vi "PH_Timing.PC link BNC Channel Infos.vi"(0 "i ref in":refnum<vi>, 1 "data":i8[](array[numeric]), 2 "Service Name":string="N/A", 3 "typeDescriptor":string="D:N", 4 "no link":bool, 5 "error in":errorcluster) -> (14 "i ref out":refnum<vi>, 19 "error out":errorcluster)   [LabVIEW 2014, in "PH_Timing.lvlib"]
doc: "This VI writes the incoming information to own attributes and sets GUI elements."
uses:
  PH_Timing.lvlib
  PH_Basics/PH_Common/PH_Common.lvlib
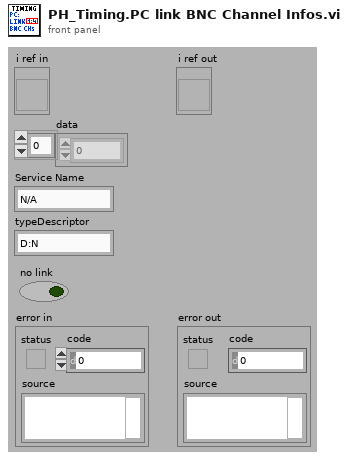
[diagram p1: front panel]
types:
  T1 = typedef "PH_Timing.lvlib/PH_Timing.i attribute.ctl" = cluster{"Sequencer":cluster{"linked?":bool, "Proc State":string, "Ref State":refnum<vi>}, "Gate Generator":cluster{"GD":cluster{"Device Status":T2, "linked?":bool}, "Settings":T3, "GUI Ref":refnum<vi>}, "Interlock Bypass":cluster{"Instancename":string, "Switch linked?":bool, "Device Status":T2, "Ref Status":refnum<vi>}, "Roughtuner":cluster{"Settings":T4, "GUI Ref":refnum<vi>, "GD":cluster{"Device Status":T2, "linked?":bool}}, "0,5Hz Gater":cluster{"Settings":T5, "GUI Ref":refnum<vi>, "GD":cluster{"Device Status":T2, "linked?":bool}}, "Slow Trigger":cluster{"Settings":T6, "GUI Ref":refnum<vi>, "Service ID Delay":i32, "Service ID Ext Trig":i32, "Wanted Settings":T6}, "Timing Mode":cluster{"Mode":T7, "GUI Ref":refnum<vi>, "Service ID T2":i32, "Service ID Mode":i32, "Wanted Mode":T7}, "ns Generator":cluster{"Settings":T8, "ns Generator Settings":refnum<vi>, "GD":cluster{"Device Status":T2, "linked?":bool}}, "Phase FEs":cluster{"Settings":T11, "GUI Ref":refnum<vi>, "Service ID Phase":i32, "Wanted Settings":T11}, "GD GUI Refs":refnum<vi>[], "Heads":T12[], "GUI Ref Delete":refnum<vi>}
  T2 = typedef "PH_StatusHandler.lvlib/PH_StatusHandler.Status.ctl" = i16
  T3 = typedef "PH_Timing.lvlib/PH_Timing.GateGen.ctl" = cluster{"Instance":string, "Channel Gate":i32, "Channel T2":i32, "Width Gate":dbl, "Width T2":dbl, "Delay Gate":dbl, "Delay T2":dbl, "Gate activ":bool, "T2 activ":bool, "System Mode":enum16{"Normal", "Single", "Burst", "Duty Cycle"}}
  T4 = typedef "PH_Timing.lvlib/PH_Timing.Roughtuner.ctl" = cluster{"Instance":string, "Phase PHELIX / UNILAC":cluster{"Channel":u16, "relative to":u16, "Delay [ms]":dbl}, "Pulse Length":cluster{"Channel":u16, "relative to":u16, "Delay [ms]":dbl}, "Trigger":cluster{"externally?":bool, "Rate [Hz]":dbl}}
  T5 = typedef "PH_Timing.lvlib/PH_Timing.0.5HzGater.ctl" = cluster{"Instance":string, "Channel ns FE Delay":i32, "Channel 0.5Hz":i32, "Width ns FE Delay":dbl, "Width 0.5Hz":dbl, "Delay ns FE Delay":dbl, "Delay 0.5Hz":dbl, "ns FE Delay active":bool, "0.5Hz activ":bool, "ns FE Delay inverted":bool, "0.5Hz inverted":bool}
  T6 = typedef "PH_Timing.lvlib/PH_Timing.Slow Trigger Settings.ctl" = cluster{"Delay":dbl, "externally triggered?":bool}
  T7 = typedef "PH_Timing.lvlib/PH_Timing.Timing Mode.ctl" = cluster{"T2":i16, "Modeselector":enum32{"10 Hz", "0.5 Hz", "Shot"}}
  T8 = typedef "PH_Timing.lvlib/PH_Timing.ns Generator.ctl" = cluster{"Instance":string, "Phase fs / ns FE":cluster{"Channel":T9, "Settings":T10}}
  T9 = typedef "Stanford Research DG645 - Driver.lvlib/Channel.ctl" = i32
  T10 = typedef "PH_SRDG645.lvlib/PH_SRDG645.Channel Settings.ctl" = cluster{"Delay [s]":dbl, "relative to":i32}
  T11 = typedef "PH_Timing.lvlib/PH_Timing.Phase FEs.ctl" = cluster{"Phase":dbl}
  T12 = typedef "PH_Timing.lvlib/PH_Timing.PU Data.ctl" = cluster{"linked?":bool, "Data":T13, "GD":cluster{"Device Status":T2, "linked?":bool}, "GUI Ref":refnum<vi>, "PU":T14}
  T13 = typedef "PH_Timing.lvlib/PH_Timing.PU Info.ctl" = cluster{"Act CH?":bool, "GD":string, "CH":i32, "Delay":dbl, "active":bool, "in Use?":bool}
  T14 = typedef "PH_PP_Common.lvlib/PH_PP_Common.PUs.ctl" = enum16{"no Info", "PA-19mm-1", "PA-19mm-2", "PA-45mm-PILC", "PA-45mm-MAIN", "MA-PU-1", "MA-PU-2", "MA-PU-3", "MA-PU-4", "MA-PU-5", "MA-PU-6", "MA-FR", "MA-PILC", "PA-45mm-DP"}
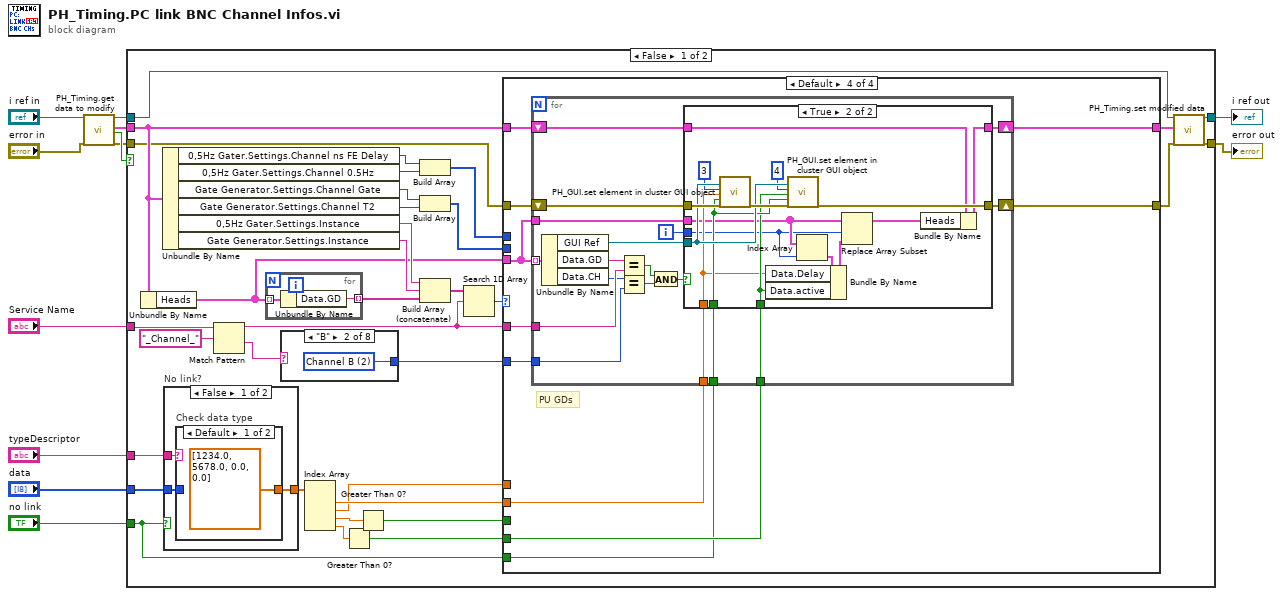
[diagram p0: block diagram]
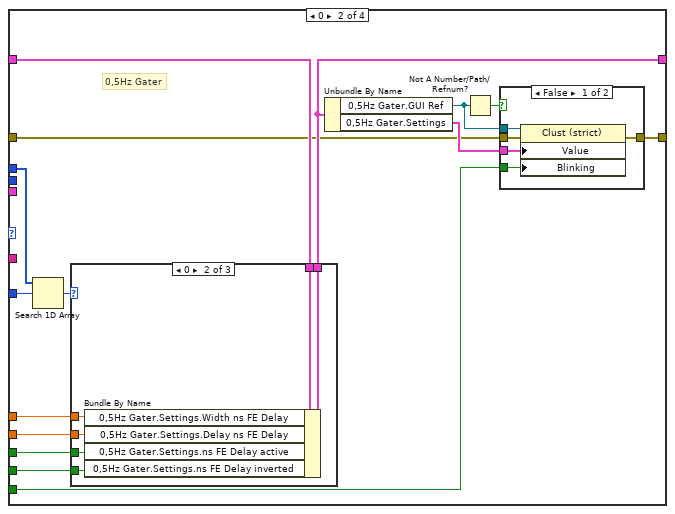
[diagram p3: hidden frame]
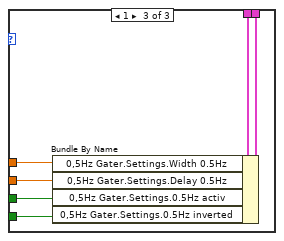
[diagram p6: hidden frame]
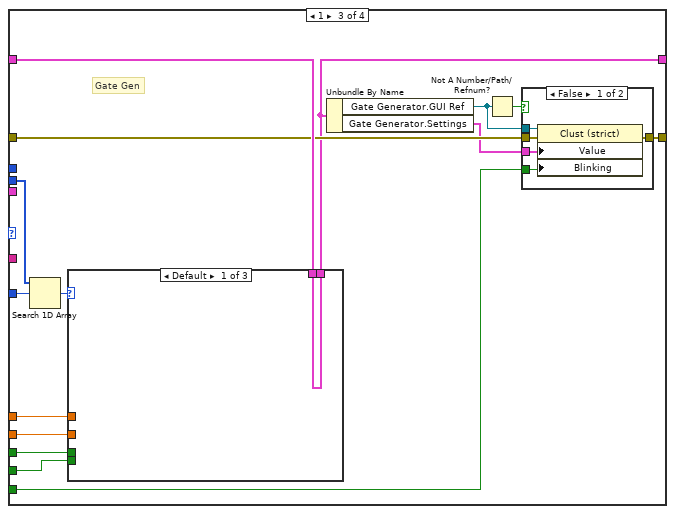
[diagram p7: hidden frame]
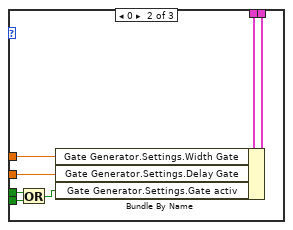
[diagram p9: hidden frame]
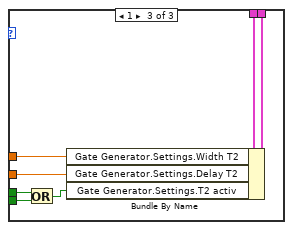
[diagram p10: hidden frame]
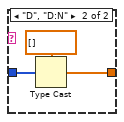
[diagram p12: hidden frame]
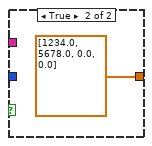
[diagram p13: hidden frame]
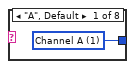
[diagram p14: hidden frame]
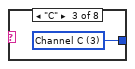
[diagram p15: hidden frame]
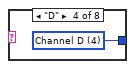
[diagram p16: hidden frame]
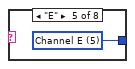
[diagram p17: hidden frame]
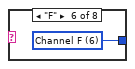
[diagram p18: hidden frame]
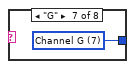
[diagram p19: hidden frame]
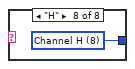
[diagram p20: hidden frame]
diagram:
  n1 = call "PH_Timing.get data to modify.vi"("i ref in"="i ref in", "error in (no error)"="error in") -> ("i ref out"=w4:refnum<vi>, "i attribute"=w9:T1, "timed out"=w10:bool, "error out"=w7:errorcluster)  [unwired: 14 in]
  n2 = case shown="False" w10 {
    tunnel: w4 -> [w16 w184]
    tunnel: [w46 w184] -> w5
    tunnel: w7 -> [w24 w183]
    tunnel: [w45 w183] -> w8
    tunnel: w9 -> [w40 _]
    tunnel: "no link" -> [w22 _]
    tunnel: "Service Name" -> [w44 _]
    tunnel: "data" -> [w33 _]
    tunnel: "typeDescriptor" -> [w32 _]
    frame False {
      n3 = Unbundle By Name(w40) -> ("Heads"=w13:T12[])
      n4 = Unbundle By Name(w40) -> ("0,5Hz Gater.Settings.Channel ns FE Delay"=w20:i32, "0,5Hz Gater.Settings.Channel 0.5Hz"=w21:i32, "Gate Generator.Settings.Channel Gate"=w37:i32, "Gate Generator.Settings.Channel T2"=w36:i32, "0,5Hz Gater.Settings.Instance"=w18:string, "Gate Generator.Settings.Instance"=w17:string)
      n5 = case "No link?" shown="False" w22 {
        tunnel: [w167 dbl[] [1234.0, 5678.0, 0.0, 0.0]] -> w31
        tunnel: w33 -> [w166 _]
        tunnel: w32 -> [w165 _]
        frame False {
          n6 = case "Check data type" shown="Default" w165 {
            tunnel: [dbl[] [1234.0, 5678.0, 0.0, 0.0] w170] -> w167
            tunnel: w166 -> [_ w171]
            frame Default {
            }
            frame "D", "D:N" {
              n7 = Type Cast(type=dbl[] [], x=w171) -> (*(type *) &x=w170:dbl[])
            }
          }
        }
        frame True {
        }
      }
      n8 = Match Pattern(string=w44, regular expression="_Channel_") -> (before substring=w15:string, after substring=w39:string)  [unwired: 1 in, 2 out]
      n9 = for {
        tunnel: w13 -> [w182] mode=indexing
        tunnel: [w181] -> w42 mode=indexing
        n10 = Unbundle By Name(w182) -> ("Data.GD"=w181:string)
      }
      n11 = case shown="\"B\"" w39 {
        tunnel: [w173 w174 w175 w176 w177 w178 w179 w180] -> w38
        frame "A", Default {
          w173 = 1 items=["System (To)", "Channel A", "Channel B", "Channel C", "Channel D", "Channel E", "Channel F", "Channel G", "Channel H"] ("Channel Gate T0")
        }
        frame "B" {
          w174 = 2 items=["System (To)", "Channel A", "Channel B", "Channel C", "Channel D", "Channel E", "Channel F", "Channel G", "Channel H"] ("Channel Gate T0")
        }
        frame "C" {
          w175 = 3 items=["System (To)", "Channel A", "Channel B", "Channel C", "Channel D", "Channel E", "Channel F", "Channel G", "Channel H"] ("Channel Gate T0")
        }
        frame "D" {
          w176 = 4 items=["System (To)", "Channel A", "Channel B", "Channel C", "Channel D", "Channel E", "Channel F", "Channel G", "Channel H"] ("Channel Gate T0")
        }
        frame "E" {
          w177 = 5 items=["System (To)", "Channel A", "Channel B", "Channel C", "Channel D", "Channel E", "Channel F", "Channel G", "Channel H"] ("Channel Gate T0")
        }
        frame "F" {
          w178 = 6 items=["System (To)", "Channel A", "Channel B", "Channel C", "Channel D", "Channel E", "Channel F", "Channel G", "Channel H"] ("Channel Gate T0")
        }
        frame "G" {
          w179 = 7 items=["System (To)", "Channel A", "Channel B", "Channel C", "Channel D", "Channel E", "Channel F", "Channel G", "Channel H"] ("Channel Gate T0")
        }
        frame "H" {
          w180 = 8 items=["System (To)", "Channel A", "Channel B", "Channel C", "Channel D", "Channel E", "Channel F", "Channel G", "Channel H"] ("Channel Gate T0")
        }
      }
      n12 = Index Array(array=w31) -> (element #1=w28:dbl, element #2=w27:dbl, element #3=w30:dbl, element #4=w29:dbl)  [unwired: 4 in]
      n13 = Greater Than 0?(x=w29) -> (x > 0?=w25:bool)
      n14 = Greater Than 0?(x=w30) -> (x > 0?=w26:bool)
      n15 = Build Array(w20, w21) -> (w19:i32[])
      n16 = Build Array(w37, w36) -> (w35:i32[])
      n17 = Build Array (concatenate)(w18, w17, w42) -> (w41:string[])
      n18 = Search 1D Array(1D array=w41, element=w15) -> (index of element=w14:i32)  [unwired: 1 in]
      n19 = case shown="Default" w14 {
        tunnel: w40 -> [w48 w63 w97 w121]
        tunnel: w35 -> [_ _ w96 _]
        tunnel: w38 -> [_ w62 w95 w127]
        tunnel: [w48 w51 w87 w120] -> w34
        tunnel: w28 -> [_ w61 w94 w124]
        tunnel: w27 -> [_ w60 w93 _]
        tunnel: w26 -> [_ w59 w92 _]
        tunnel: w25 -> [_ w58 w91 w123]
        tunnel: w24 -> [w47 w50 w89 w126]
        tunnel: [w47 w49 w88 w125] -> w23
        tunnel: w13 -> [_ _ _ w119]
        tunnel: w15 -> [_ _ _ w128]
        tunnel: w22 -> [_ w52 w86 w122]
        tunnel: w19 -> [_ w56 _ _]
        frame -1 {
        }
        frame 0 {
          # "0,5Hz Gater"
          n20 = Search 1D Array(1D array=w56, element=w62) -> (index of element=w57:i32)  [unwired: 1 in]
          n21 = case shown="0" w57 {
            tunnel: w63 -> [w70 w76 w82]
            tunnel: [w70 w75 w81] -> w51
            tunnel: w61 -> [_ w73 w79]
            tunnel: w60 -> [_ w74 w80]
            tunnel: w59 -> [_ w72 w78]
            tunnel: w58 -> [_ w71 w77]
            frame -1, Default {
            }
            frame 0 {
              n22 = Bundle By Name(cluster=w76, "0,5Hz Gater.Settings.Width ns FE Delay"=w74, "0,5Hz Gater.Settings.Delay ns FE Delay"=w73, "0,5Hz Gater.Settings.ns FE Delay active"=w72, "0,5Hz Gater.Settings.ns FE Delay inverted"=w71) -> (w75:T1)
            }
            frame 1 {
              n23 = Bundle By Name(cluster=w82, "0,5Hz Gater.Settings.Width 0.5Hz"=w80, "0,5Hz Gater.Settings.Delay 0.5Hz"=w79, "0,5Hz Gater.Settings.0.5Hz activ"=w78, "0,5Hz Gater.Settings.0.5Hz inverted"=w77) -> (w81:T1)
            }
          }
          n24 = Unbundle By Name(w51) -> ("0,5Hz Gater.GUI Ref"=w53:refnum<vi>, "0,5Hz Gater.Settings"=w55:T5)
          n25 = Not A Number/Path/Refnum?(number/path/refnum=w53) -> (NaN/Path/Refnum?=w54:bool)
          n26 = case shown="False" w54 {
            tunnel: [w68 w69] -> w49
            tunnel: w53 -> [w67 _]
            tunnel: w55 -> [w66 _]
            tunnel: w52 -> [w65 _]
            tunnel: w50 -> [w64 w69]
            frame False {
              n27 = property class="Clust (strict)"(reference=w67, error in=w64, "Value"=w66, "Blinking"=w65) -> (error out=w68:errorcluster)  [unwired: 1 out]
            }
            frame True {
            }
          }
        }
        frame 1 {
          # "Gate Gen"
          n28 = Search 1D Array(1D array=w96, element=w95) -> (index of element=w90:i32)  [unwired: 1 in]
          n29 = case shown="Default" w90 {
            tunnel: w97 -> [w104 w111 w118]
            tunnel: [w104 w110 w117] -> w87
            tunnel: w94 -> [_ w106 w116]
            tunnel: w93 -> [_ w109 w115]
            tunnel: w92 -> [_ w108 w114]
            tunnel: w91 -> [_ w107 w113]
            frame Default {
            }
            frame 0 {
              n30 = Or(x=w108, y=w107) -> (x .or. y?=w105:bool)
              n31 = Bundle By Name(cluster=w111, "Gate Generator.Settings.Width Gate"=w109, "Gate Generator.Settings.Delay Gate"=w106, "Gate Generator.Settings.Gate activ"=w105) -> (w110:T1)
            }
            frame 1 {
              n32 = Or(x=w114, y=w113) -> (x .or. y?=w112:bool)
              n33 = Bundle By Name(cluster=w118, "Gate Generator.Settings.Width T2"=w115, "Gate Generator.Settings.Delay T2"=w116, "Gate Generator.Settings.T2 activ"=w112) -> (w117:T1)
            }
          }
          n34 = Unbundle By Name(w87) -> ("Gate Generator.GUI Ref"=w83:refnum<vi>, "Gate Generator.Settings"=w85:T3)
          n35 = Not A Number/Path/Refnum?(number/path/refnum=w83) -> (NaN/Path/Refnum?=w84:bool)
          n36 = case shown="False" w84 {
            tunnel: w89 -> [w102 w103]
            tunnel: [w101 w103] -> w88
            tunnel: w83 -> [w100 _]
            tunnel: w86 -> [w99 _]
            tunnel: w85 -> [w98 _]
            frame False {
              n37 = property class="Clust (strict)"(reference=w100, error in=w102, "Value"=w98, "Blinking"=w99) -> (error out=w101:errorcluster)  [unwired: 1 out]
            }
            frame True {
            }
          }
        }
        frame Default {
          # "PU GDs"
          n38 = for {
            tunnel: w119 -> [w131] mode=indexing
            tunnel: w128 -> [w145]
            tunnel: w127 -> [w144]
            shift-right: [w139] -> w125
            shift-left: w126 -> [w140]
            tunnel: w124 -> [w136]
            tunnel: w123 -> [w135]
            tunnel: w122 -> [w134]
            shift-right: [w132] -> w120
            shift-left: w121 -> [w133]
            tunnel: w119 -> [w130]
            i -> [w129]
            n39 = Unbundle By Name(w131) -> ("GUI Ref"=w137:refnum<vi>, "Data.GD"=w146:string, "Data.CH"=w143:i32)
            n40 = Equal?(x=w146, y=w145) -> (x = y?=w141:bool)
            n41 = Equal?(x=w143, y=w144) -> (x = y?=w142:bool)
            n42 = And(x=w141, y=w142) -> (x .and. y?=w138:bool)
            n43 = case shown="True" w138 {
              tunnel: w140 -> [w148 w164]
              tunnel: [w148 w162] -> w139
              tunnel: w137 -> [_ w161]
              tunnel: w136 -> [_ w154]
              tunnel: w135 -> [_ w155]
              tunnel: w134 -> [_ w160]
              tunnel: [w147 w157] -> w132
              tunnel: w133 -> [w147 w156]
              tunnel: w130 -> [_ w152]
              tunnel: w129 -> [_ w150]
              frame False {
              }
              frame True {
                n44 = call "PH_GUI.set element in cluster GUI object.vi"("Cluster Ref"=w161, "Cluster index"=3, "Value"=w154, "Blinking? (false)"=w160, "error in (no error)"=w164) -> ("error out"=w163:errorcluster)  [unwired: 14 in]
                n45 = call "PH_GUI.set element in cluster GUI object.vi"("Cluster Ref"=w161, "Cluster index"=4, "Value"=w155, "Blinking? (false)"=w160, "error in (no error)"=w163) -> ("error out"=w162:errorcluster)  [unwired: 14 in]
                n46 = Index Array(array=w152, index=w150) -> (element=w151:T12)
                n47 = Bundle By Name(cluster=w151, "Data.Delay"=w154, "Data.active"=w155) -> (w153:T12)
                n48 = Replace Array Subset(array=w152, new element=w153, index=w150) -> (w149:T12[])
                n49 = Bundle By Name(cluster=w156, "Heads"=w149) -> (w157:T1)
              }
            }
          }
        }
      }
      n50 = call "PH_Timing.set modified data.vi"("i ref in"=w16, "i attribute"=w34, "error in (no error)"=w23) -> ("i ref out"=w46:refnum<vi>, "error out"=w45:errorcluster)  [unwired: 15 in]
    }
    frame True {
      (unwired) -1 ("index of element")
    }
  }
  "error out" <- w8
  "i ref out" <- w5
